vi "test-NameMap.vi"() -> ()   [LabVIEW 2019, in "lv-apt-json-file-test.lvlib"]
uses:
  lv-apt-json-file-test.lvlib
  Typedef/Def-NameMap.ctl
  lv-apt-json-file.lvlib
panel:
  out "OriginName":string
  out "NameMap out":T1
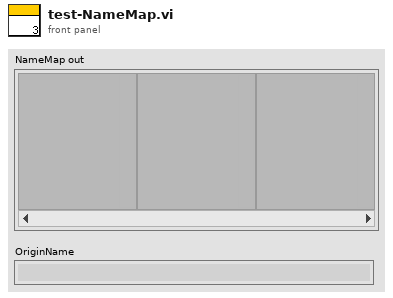
[diagram p1: front panel]
types:
  T1 = typedef "lv-apt-json-file.lvlib/Def-NameMap.ctl" = variant[]
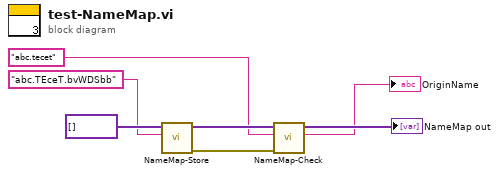
[diagram p0: block diagram]
diagram:
  n1 = call "NameMap-Store.vi"("name"="abc.TEceT.bvWDSbb", "NameMap in"=T1 []) -> ("error out"=w1:errorcluster, "NameMap out"=w5:T1)  [unwired: 8 in]
  n2 = call "NameMap-Check.vi"("error in (no error)"=w1, "Name"="abc.tecet", "NameMap in"=w5) -> ("OriginName"=→"OriginName":string, "NameMap out"=→"NameMap out":T1)  [unwired: 6 in, 1 out]
